vi "setUp.vi"(8 "error in (no error)":errorcluster, 11 "reference in":refnum<class "Parameter Setting.lvclass">) -> (0 "error out":errorcluster, 3 "reference out":refnum<class "Parameter Setting.lvclass">)   [LabVIEW 2017, in "Deterministic Error Tests.lvlib" / "Parameter Setting.lvclass"]
doc: "setUp runs prior to the test method during test execution. Use this method to initialize any object data required by your tests."
uses:
  Parameter Setting.lvclass
  C:/Program Files (x86)/National Instruments/LabVIEW 2017/vi.lib/addons/_JKI Toolkits/VI Tester/TestCase.llb/TestCase.lvclass
  Parameter Setting.lvclass/Parameter Setting.ctl
  Source/VIs/VIs for Poly/Create Error Cluster (256B).vi
  <vilib>/addons/_JKI Toolkits/VI Tester/TestCase.llb/TestCase.lvclass
  Source/Deterministic Error Builder.lvlib
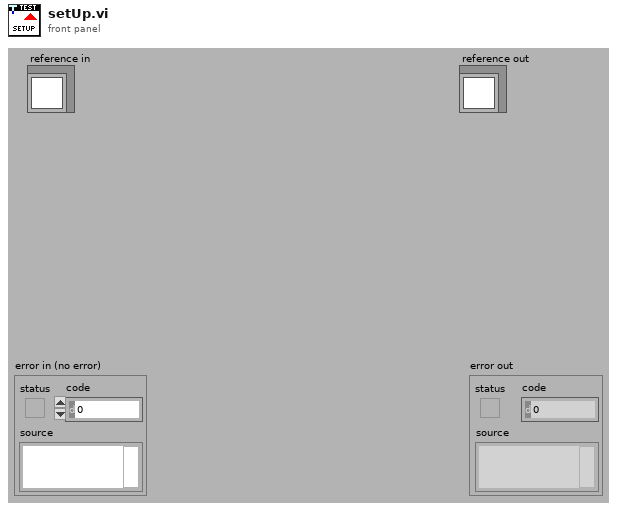
[diagram p1: front panel]
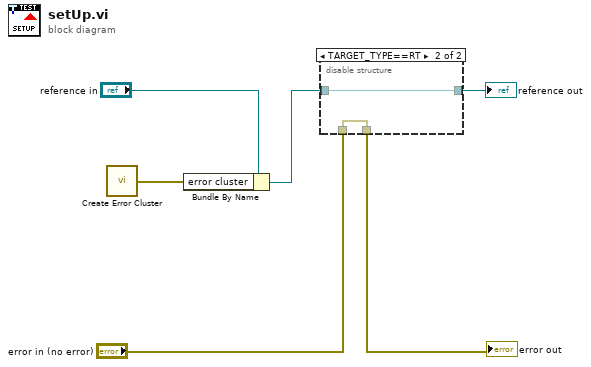
[diagram p0: block diagram]
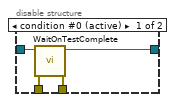
[diagram p2: hidden frame]
diagram:
  n1 = call-poly "Create Error Cluster.vi"() -> ("error out"=w1:errorcluster)  [unwired: 1 in]
  n2 = Bundle By Name(cluster="reference in", "error cluster"=w1) -> (w2:refnum<class "Parameter Setting.lvclass">)
  n3 = disable-structure shown="TARGET_TYPE==RT" {
    disable-tunnel: "error in (no error)" -> [w10 w11]
    disable-tunnel: [w9 w11] -> w5
    disable-tunnel: [w8 w12] -> w3
    disable-tunnel: w2 -> [w7 w12]
    frame condition #0 (active) {
      n4 = call <vilib>:"WaitOnTestComplete.vi"("error in (no error)"=w10, "TestCase in"=w7) -> ("error out"=w9:errorcluster, "TestCase out"=w8:refnum<class "Parameter Setting.lvclass">)  [unwired: 8 in]
    }
    frame condition #1 {
    }
  }
  "error out" <- w5
  "reference out" <- w3
